vi "Create Virtual Folder (Target In).vi"(8 "error in":errorcluster, 10 "Item to Find":string, 11 "TargetItem in":refnum<vi>) -> (0 "error out":errorcluster, 3 "ProjectItem out":refnum<vi>)   [LabVIEW 2014, in "SPI Engine Scripting.lvlib"]
uses:
  SPI Engine Scripting.lvlib
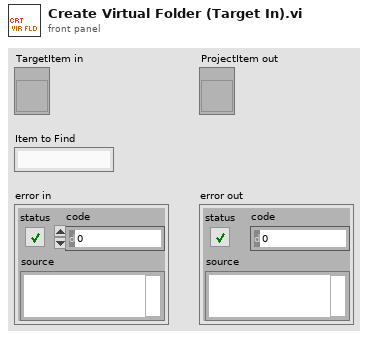
[diagram p1: front panel]
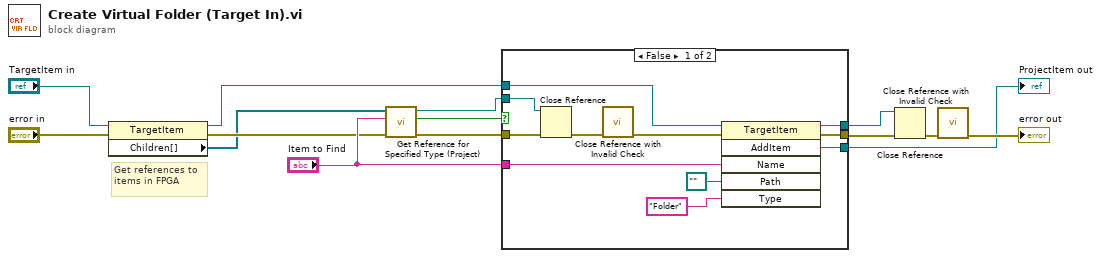
[diagram p0: block diagram]
diagram:
  # "Get references to items in FPGA"
  n1 = property class="TargetItem"(reference="TargetItem in", error in="error in") -> (reference out=w6:refnum<vi>, error out=w5:errorcluster, "Children[]"=w1:refnum<vi>[])
  n2 = call "Get Reference for Specified Type (Project).vi"("error in (no error)"=w5, "Type to Find"="Item to Find", "Array of References"=w1) -> ("error out"=w3:errorcluster, "Item Found"=w2:bool, "Project Item"=w4:refnum<vi>)  [unwired: 6 in]
  n3 = case shown="False" w2 {
    tunnel: [w25 w27] -> w10
    tunnel: w3 -> [w17 w28]
    tunnel: w4 -> [w16 w27]
    tunnel: [w20 w28] -> w11
    tunnel: w6 -> [w22 w26]
    tunnel: "Item to Find" -> [w21 _]
    tunnel: [w19 w26] -> w14
    frame False {
      n4 = Close Reference(reference=w16, error in (no error)=w17) -> (error out=w18:errorcluster)
      n5 = call "Close Reference with Invalid Check.vi"("error in (no error)"=w18) -> ("error out"=w15:errorcluster)  [unwired: 10 in]
      n6 = invoke class="TargetItem" method="AddItem"(reference=w22, error in=w15, "Name"=w21, "Path"=path "", "Type"="Folder") -> (reference out=w19:refnum<vi>, error out=w20:errorcluster, "AddItem"=w25:refnum<vi>)  [unwired: 1 in, 3 out]
    }
    frame True {
    }
  }
  "ProjectItem out" <- w10
  n7 = Close Reference(reference=w14, error in (no error)=w11) -> (error out=w12:errorcluster)
  n8 = call "Close Reference with Invalid Check.vi"("error in (no error)"=w12) -> ("error out"=→"error out":errorcluster)  [unwired: 10 in]
